vi "cycle_read.vi"() -> ()   [LabVIEW 2014]
uses:
  Robot_Position.ctl
  <vilib>/Tufts CEEO ROS for LabVIEW Software/ROS/Code/Console/Servers/ServerSubs/TopicDef.ctl
  <vilib>/Tufts CEEO ROS for LabVIEW Software/ROS/Code/SubVIs/_ROSDirection.ctl
panel:
  out "错误输出":errorcluster
  out "sensor_msg_cluster":cluster{"voltage":dbl, "motor":i8}
  out "robot_position_cluster":T1
  in  "stop2":bool
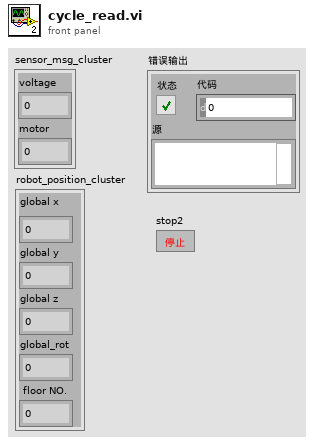
[diagram p1: front panel]
types:
  T1 = typedef "Robot_Position.ctl" = cluster{"global x":dbl, "global y":dbl, "global z":dbl, "global_rot":dbl, " floor NO.":dbl}
  T2 = typedef "TopicDef.ctl" = cluster{"Topic":string, "Type":string, "Action":T3, "Update (ms)":u16, "queue size":u16}
  T3 = typedef "_ROSDirection.ctl" = enum16{"Node", "Publisher", "Subscriber", "ServiceClient", "ServiceProvider"}
  T4 = typedef "_ROSControl.ctl" = cluster{"topic port":u16, "Node":string, "topic":string, "type":string, "node port":u16, "error ":errorcluster, "Direction":T3, "Update (ms)":u16, "FIFO size":u16}
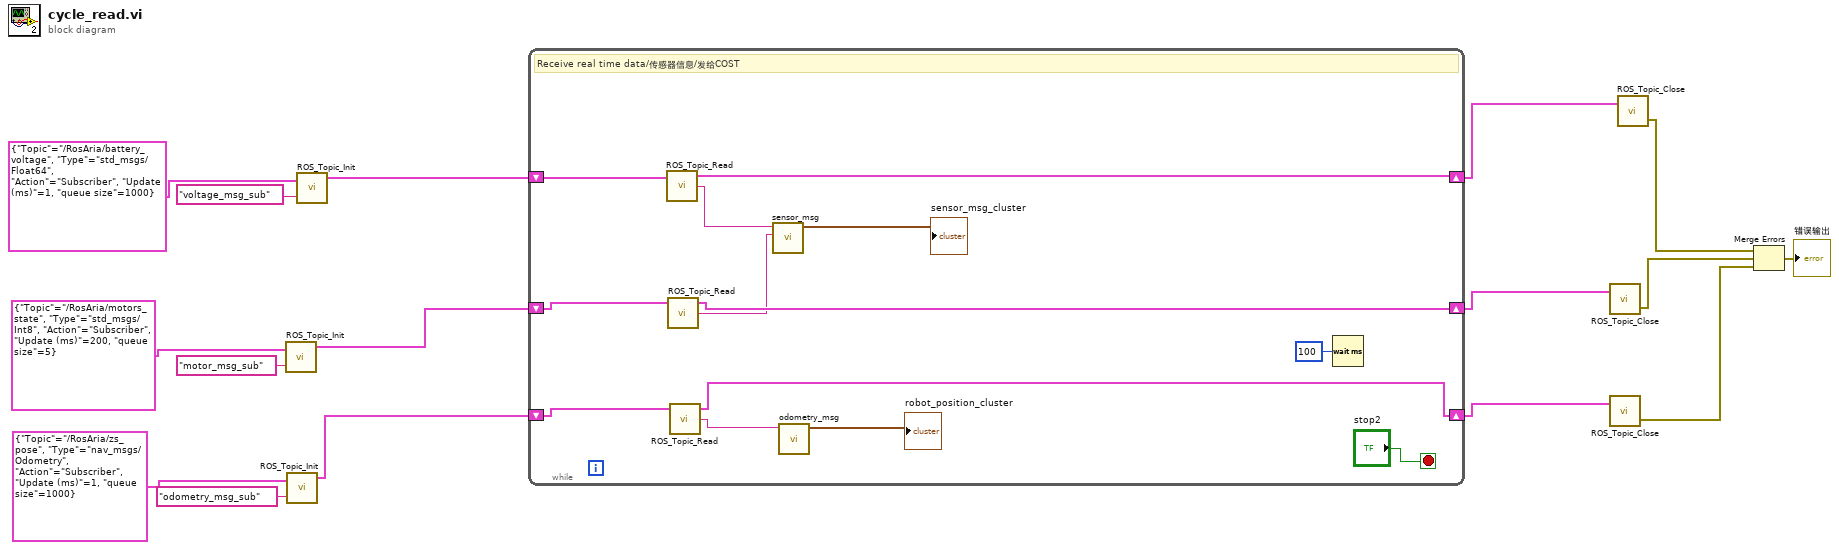
[diagram p0: block diagram]
diagram:
  n1 = call <vilib>:"ROS_Topic_Init.vi"("Definitions"=T2 {"Topic"="/RosAria/motors_state", "Type"="std_msgs/Int8", "Action"=enum."Subscriber", "Update (ms)"=200, "queue size"=5}, "node"="motor_msg_sub") -> ("ROS out"=w10:T4)  [unwired: 1 in, 1 out]
  n2 = call <vilib>:"ROS_Topic_Init.vi"("Definitions"=T2 {"Topic"="/RosAria/zs_pose", "Type"="nav_msgs/Odometry", "Action"=enum."Subscriber", "Update (ms)"=1, "queue size"=1000}, "node"="odometry_msg_sub") -> ("ROS out"=w6:T4)  [unwired: 1 in, 1 out]
  n3 = call <vilib>:"ROS_Topic_Init.vi"("Definitions"=T2 {"Topic"="/RosAria/battery_voltage", "Type"="std_msgs/Float64", "Action"=enum."Subscriber", "Update (ms)"=1, "queue size"=1000}, "node"="voltage_msg_sub") -> ("ROS out"=w12:T4)  [unwired: 1 in, 1 out]
  n4 = while {
    shift-right: [w27] -> w11
    shift-left: w12 -> [w28]
    shift-right: [w25] -> w9
    shift-left: w10 -> [w26]
    shift-right: [w23] -> w5
    shift-left: w6 -> [w24]
    stop <- "stop2" stop-if-true
    # "Receive real time data/传感器信息/发给COST"
    n5 = call <vilib>:"ROS_Topic_Read.vi"("ROS in"=w28) -> ("Reply"=w22:string, "ROS out"=w27:T4)  [unwired: 2 in, 1 out]
    n6 = call <vilib>:"ROS_Topic_Read.vi"("ROS in"=w26) -> ("Reply"=w21:string, "ROS out"=w25:T4)  [unwired: 2 in, 1 out]
    n7 = call <vilib>:"ROS_Topic_Read.vi"("ROS in"=w24) -> ("Reply"=w20:string, "ROS out"=w23:T4)  [unwired: 2 in, 1 out]
    n8 = call "sensor_msg.vi"("motor_msg in"=w21, "voltage_msg in"=w22) -> ("sensor_msg_cluster"=→"sensor_msg_cluster":cluster{"voltage":dbl, "motor":i8})  [unwired: 9 in]
    n9 = call "odometry_msg.vi"("odometry_msg in"=w20) -> ("robot_position_cluster"=→"robot_position_cluster":T1)  [unwired: 9 in, 1 out]
    n10 = Wait (ms)(milliseconds to wait=u32 100 ("等待时间（毫秒）")) -> ()  [unwired: 1 out]
  }
  n11 = call <vilib>:"ROS_Topic_Close.vi"("ROS in"=w9) -> ("error out"=w3:errorcluster)  [unwired: 3 in]
  n12 = call <vilib>:"ROS_Topic_Close.vi"("ROS in"=w5) -> ("error out"=w2:errorcluster)  [unwired: 3 in]
  n13 = call <vilib>:"ROS_Topic_Close.vi"("ROS in"=w11) -> ("error out"=w4:errorcluster)  [unwired: 3 in]
  n14 = Merge Errors(w4, w3, w2) -> (→"错误输出":errorcluster)
